vi "Sanitize input.vi"(11 "TipTable":T1) -> (2 "valid?":bool, 3 "TipTable":T1)   [LabVIEW 2021, in "RocketPlot.lvlib" / "TipTablePanel.lvclass"]
uses:
  TipTablePanel.lvclass
  new tip instructions.ctl
  cell cache.ctl
  colors.ctl
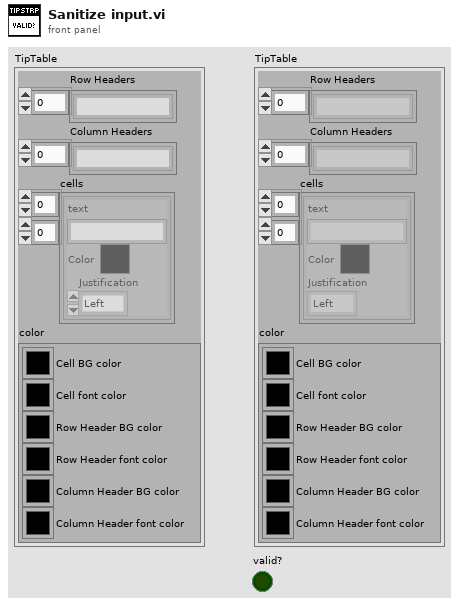
[diagram p1: front panel]
types:
  T1 = typedef "RocketPlot.lvlib/TipTablePanel.lvclass/new tip instructions.ctl" = cluster{"Row Headers":string[], "Column Headers":string[], "cells":T2[][], "color":T3}
  T2 = typedef "RocketPlot.lvlib/TipTablePanel.lvclass/cell cache.ctl" = cluster{"text":string, "Color":u32, "Justification":enum16{"Left", "Center", "Right"}}
  T3 = typedef "RocketPlot.lvlib/TipTablePanel.lvclass/colors.ctl" = cluster{"Cell BG color":u32, "Cell font color":u32, "Row Header BG color":u32, "Row Header font color":u32, "Column Header BG color":u32, "Column Header font color":u32}
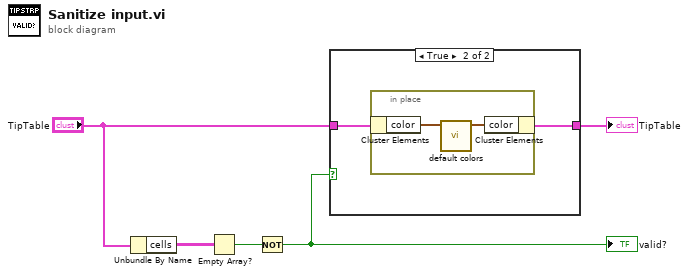
[diagram p0: block diagram]
diagram:
  n1 = Unbundle By Name("TipTable") -> ("cells"=w3:T2[][])
  n2 = Empty Array?(array=w3) -> (empty?=w2:bool)
  n3 = Not(x=w2) -> (.not. x?=w1:bool)
  "valid?" <- w1
  n4 = case shown="True" w1 {
    tunnel: [_ w7] -> w5
    tunnel: "TipTable" -> [_ w6]
    frame False {
    }
    frame True {
      n5 = in-place {
        n6 = in-place-cluster #1(w6) -> ("color"=w9:T3)
        n7 = call "default colors.vi"("colors"=w9) -> ("default color"=w8:T3)  [unwired: 10 in]
        n8 = in-place-cluster #1("color"=w8) -> (w7:T1)
      }
    }
  }
  "TipTable" <- w5
